vi "IMAQCalculateFPS.vi"(2 "Update interval":u32=1000, 3 "buffer number":u32) -> (0 "processed FPS":dbl, 1 "acquired FPS":dbl)   [LabVIEW 2012, in "HGF_VisionTools.lvlib"]
doc: "Calculate the frame rate from within a loop. Frame rate is averaged over the specified update interval. The default update interval is 1000ms."
uses:
  HGF_VisionTools.lvlib
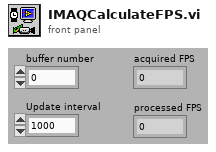
[diagram p1: front panel]
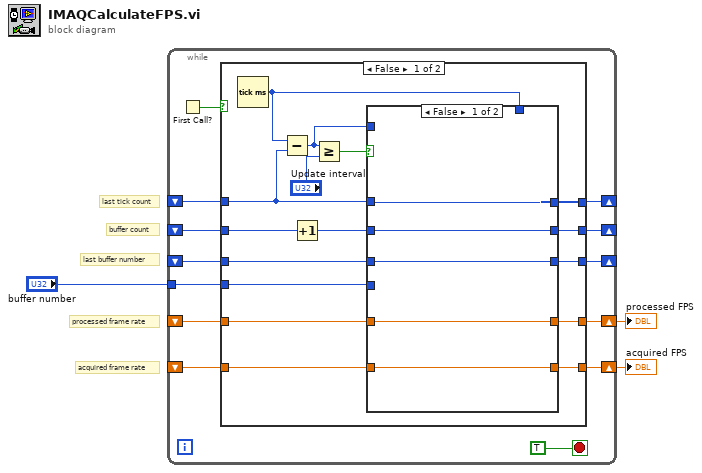
[diagram p0: block diagram]
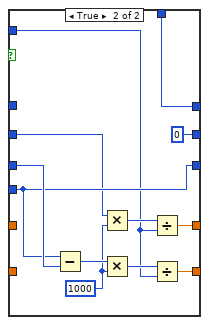
[diagram p2: hidden frame]
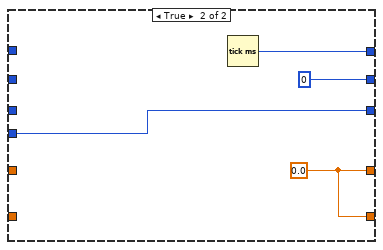
[diagram p3: hidden frame]
diagram:
  # "processed frame rate"
  # "buffer count"
  # "last buffer number"
  # "acquired frame rate"
  # "last tick count"
  n1 = while {
    shift-right: [w14] -> _
    shift-left: _ -> [w13]
    shift-right: [w11] -> _
    shift-left: _ -> [w12]
    shift-right: [w10] -> w3
    shift-left: _ -> [w9]
    tunnel: "buffer number" -> [w8]
    shift-right: [w7] -> _
    shift-left: _ -> [w6]
    shift-right: [w5] -> w1
    shift-left: _ -> [w4]
    stop <- TRUE stop-if-true
    n2 = First Call?() -> (First Call?: T/F=w15:bool)
    n3 = case shown="False" w15 {
      tunnel: [w29 w53] -> w14
      tunnel: w13 -> [w30 _]
      tunnel: w12 -> [w28 _]
      tunnel: [w27 w52] -> w11
      tunnel: [w24 w50] -> w10
      tunnel: w9 -> [w23 _]
      tunnel: w8 -> [w22 w52]
      tunnel: [w21 u32 0 ("buffer number")] -> w7
      tunnel: w6 -> [w18 _]
      tunnel: [w20 w50] -> w5
      tunnel: w4 -> [w19 _]
      frame False {
        n4 = Tick Count (ms)() -> (millisecond timer value=w26:u32)
        n5 = Subtract(x=w26, y=w30) -> (x-y=w25:u32)
        n6 = Increment(x=w18) -> (x+1=w17:u32)
        n7 = Greater Or Equal?(x=w25, y="Update interval") -> (x >= y?=w31:bool)
        n8 = case shown="False" w31 {
          tunnel: w30 -> [w37 _]
          tunnel: [w37 w49] -> w29
          tunnel: w28 -> [w35 w45]
          tunnel: [w35 w44] -> w27
          tunnel: w26 -> [_ w49]
          tunnel: w25 -> [_ w39]
          tunnel: [w36 w47] -> w24
          tunnel: w23 -> [w36 _]
          tunnel: w22 -> [_ w44]
          tunnel: w17 -> [w33 w41]
          tunnel: [w33 u32 0] -> w21
          tunnel: [w34 w38] -> w20
          tunnel: w19 -> [w34 _]
          frame False {
          }
          frame True {
            w42 = u32 1000 ("y")
            n9 = Subtract(x=w44, y=w45) -> (x-y=w46:u32)
            n10 = Multiply(x=w41, y=w42) -> (x*y=w40:u32)
            n11 = Multiply(x=w46, y=w42) -> (x*y=w48:u32)
            n12 = Divide(x=w40, y=w39) -> (x/y=w38:dbl)
            n13 = Divide(x=w48, y=w39) -> (x/y=w47:dbl)
          }
        }
      }
      frame True {
        w50 = 0.0
        n14 = Tick Count (ms)() -> (millisecond timer value=w53:u32)
      }
    }
  }
  "acquired FPS" <- w3
  "processed FPS" <- w1
